vi "Simple Serial Test.vi"() -> ()   [LabVIEW 2018]
doc: "This example performs a serial port write and a serial port read. The parameters set for the serial port must match the parameters of the connected instrument or device. The VISA Configure Serial Port VI sets the configuration parameters. The front panel displays the controls used to configure the basic parameters, such as baud rate, data bits, and parity. The VI passes the VISA resource name to other VIs that perform operations on that VISA resource. The VISA Write function sends a command to the serial device and the VISA Read function returns data based on the command. The VISA Close function then closes the reference to the serial device. It is important to close the reference; otherwise, further communication through that port might not be possible."
uses:
  Program Files/National Instruments/LabVIEW 2018/examples/Instrument IO/Serial/support/Serial - Settings.ctl
  <vilib>/Instr/_visa.llb/VISA Configure Serial Port (Instr).vi
  Hitronics.lvclass
panel:
  out "number":u32
  in  "Command":string="ªU\u0000\u0004€„"
  in  "Serial Settings":T1={"baud rate"=115200, "data bits"=8, "parity"=enum."None", "stop bits"=10, "flow control"=0} {"flow control" items=["None"=0, "XON/XOFF"=1, "RTS/CTS"=2, "DTR/DSR"=4]; "stop bits" items=["1.0"=10, "1.5"=15, "2.0"=20]; "data bits" min=5 max=8 step=1; "baud rate" items=["75"=75, "110"=110, "134"=134, "150"=150, "300"=300, "600"=600, "1200"=1200, "1800"=1800, "2400"=2400, "4800"=4800, "7200"=7200, "9600"=9600, "14400"=14400, "19200"=19200, "28800"=28800, "38400"=38400, "56000"=56000, "57600"=57600, "115200"=115200, "128000"=128000, "230400"=230400]}
  out "bytes read":u32
  in  "delay before read (ms)":u32=500
  out "Response":string
  in  "VISA resource name":refnum<visa-resource-name>="COM1"
  # "Overview: Demonstrates the use of the VISA functions to send a single command to a serial instrument and read a response.\nRequirements: NI-VISA Driver\nInstructions:\n1. Ensure the resource specified by the VISA resource name is a valid serial device.\n2. Run the VI.\n3. If your instrument recognizes the \"*IDN?\" command, it should return a Response."
  # "Note: For an example of how to perform continuous serial communication in a loop, open the Continuous Serial Write and Read.vi in the same folder as this example."
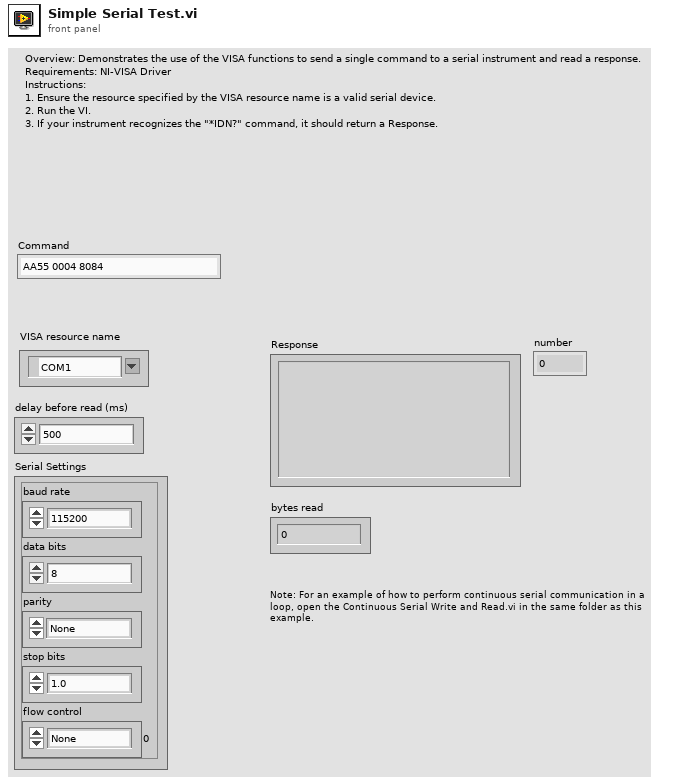
[diagram p1: front panel]
types:
  T1 = typedef "Hitronics.lvlib/Hitronics.lvclass/Serial - Settings.ctl" = cluster{"baud rate":u32, "data bits":u16, "parity":enum16{"None", "Odd", "Even", "Mark", "Space"}, "stop bits":u16, "flow control":u16}
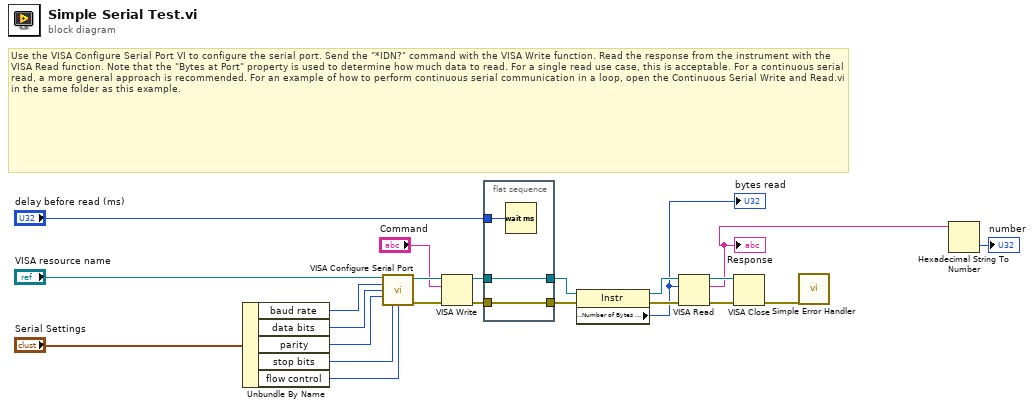
[diagram p0: block diagram]
diagram:
  # "Use the VISA Configure Serial Port VI to configure the serial port. Send the \"*IDN?\" command with the VISA Write function. Read the response from the instrument with the VISA Read function. Note that the \"Bytes at Port\" property is used to determine how much data to read. For a single read use case, this is acceptable. For a continuous serial read, a more general approach is recommended. For an example of how to perform continuous serial communication in a loop, open the Continuous Serial Write and Read.vi in the same folder as this example."
  n1 = Unbundle By Name("Serial Settings") -> ("baud rate"=w7:u32, "data bits"=w6:u16, "parity"=w5:enum16{"None", "Odd", "Even", "Mark", "Space"}, "stop bits"=w4:u16, "flow control"=w3:u16)
  n2 = call-poly "VISA Configure Serial Port"("VISA resource name"="VISA resource name", "baud rate (9600)"=w7, "data bits (8)"=w6, "parity (0:none)"=w5, "stop bits (10: 1 bit)"=w4, "flow control (0:none)"=w3) -> ("VISA resource name out"=w21:refnum<visa-resource-name>, "error out"=w22:errorcluster)  [unwired: 3 in, 5 out]
  n3 = VISA Write(VISA resource name=w21, write buffer="Command", error in (no error)=w22) -> (VISA resource name out=w15:refnum<visa-resource-name>, error out=w17:errorcluster)  [unwired: 1 out]
  n4 = flat-sequence {
    tunnel: w17 -> [w25]
    tunnel: [w25] -> w16
    tunnel: w15 -> [w24]
    tunnel: [w24] -> w14
    tunnel: "delay before read (ms)" -> [w26]
    frame #0 {
      n5 = Wait (ms)(milliseconds to wait=w26) -> ()  [unwired: 1 out]
    }
  }
  n6 = property class="Instr"(reference=w14, error in=w16) -> (reference out=w11:refnum<visa-resource-name>, error out=w10:errorcluster, "Serial Settings:Number of Bytes at Serial Port"=w9:u32)
  "bytes read" <- w9
  n7 = VISA Read(VISA resource name=w11, byte count=w9, error in (no error)=w10) -> (VISA resource name out=w19:refnum<visa-resource-name>, read buffer=w2:string, error out=w20:errorcluster)  [unwired: 1 out]
  "Response" <- w2
  n8 = VISA Close(VISA resource name=w19, error in (no error)=w20) -> (error out=w18:errorcluster)
  n9 = call <vilib>:"Simple Error Handler.vi"("error in (no error)"=w18) -> ()  [unwired: 1 in, 8 out]
  n10 = Hexadecimal String To Number(string=w2) -> (number=→"number":u32)  [unwired: 2 in, 1 out]
